vi "Actualiza Tabla.vi"(8 "error in (no error)":errorcluster, 10 "ACTUALIZA TABLA":bool, 11 "CAFE ACTOR in":refnum<class "CAFE ACTOR.lvclass">) -> (0 "error out":errorcluster, 3 "CAFE ACTOR out":refnum<class "CAFE ACTOR.lvclass">)   [LabVIEW 2019, in "CAFE ACTOR.lvlib" / "CAFE ACTOR.lvclass"]
uses:
  CAFE ACTOR.lvclass
  CAFE ACTOR.lvclass/CAFE ACTOR.ctl
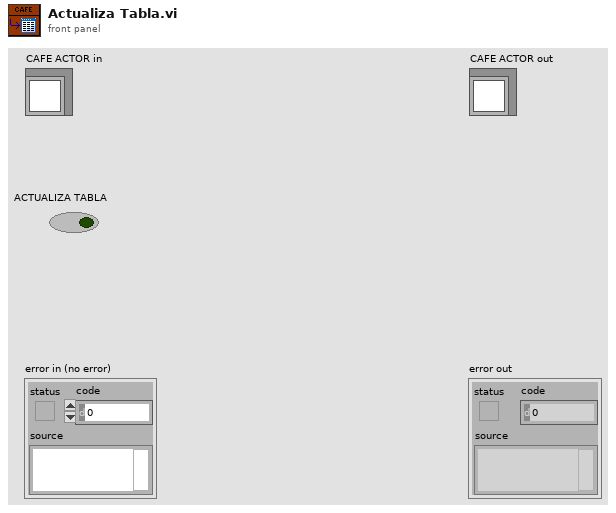
[diagram p1: front panel]
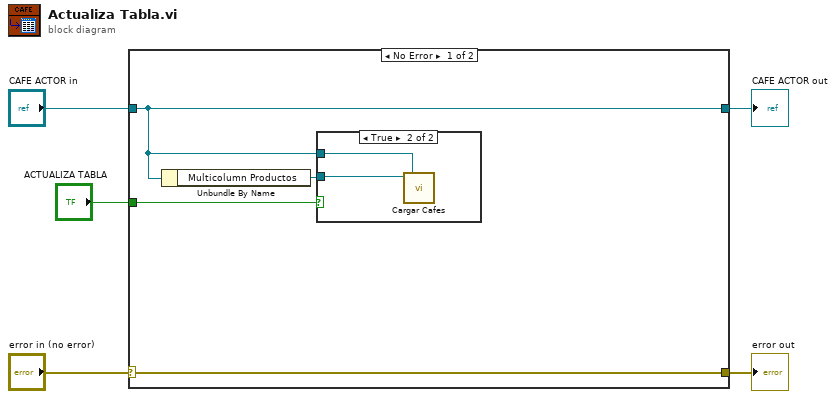
[diagram p0: block diagram]
diagram:
  n1 = case shown="No Error" "error in (no error)" {
    selector: "error in (no error)" -> [w9 w13]
    tunnel: [w9 w13] -> w2
    tunnel: [w6 w12] -> w1
    tunnel: "CAFE ACTOR in" -> [w6 w12]
    tunnel: "ACTUALIZA TABLA" -> [w8 _]
    frame No Error {
      n2 = Unbundle By Name(w6) -> ("Multicolumn Productos"=w7:refnum<vi>)
      n3 = case shown="True" w8 {
        tunnel: w7 -> [_ w10]
        tunnel: w6 -> [_ w11]
        frame False {
        }
        frame True {
          n4 = call "Cargar Cafes.vi"("CAFE ACTOR in"=w11, "MulticolumnListbox in"=w10) -> ()  [unwired: 10 in]
        }
      }
    }
    frame Error {
    }
  }
  "error out" <- w2
  "CAFE ACTOR out" <- w1
